vi "AO DM setup.vi"() -> ()   [LabVIEW 2018]
uses:
  <userlib>/WaveKit.lib/Controls/Wavefront Corrector states - ONE.ctl
  <userlib>/WaveKit.lib/Classes/WavefrontCorrector/WavefrontCorrector.lvclass
  <userlib>/WaveKit.lib/Classes/WavefrontCorrectorSet/WavefrontCorrectorSet.lvclass
  <vilib>/Utility/file.llb/Read From Spreadsheet File (DBL).vi
  <vilib>/Analysis/1siggen.llb/Ramp Pattern by Delta.vi
  <userlib>/WaveKit.lib/Classes/ModalCoef/ModalCoef.lvclass
  <userlib>/WaveKit.lib/Controls/Pupil.lvclass
  <vilib>/Analysis/NI_AALBase.lvlib
panel:
  out "DM Status":sgl[](graph)
  in  "SaveFile":bool=TRUE
  in  "Output folder":path=path "D:/Data"
  in  "File prefix name":string="Test"
  out "Final Positions":sgl[](array[numeric])
  out "Zern coef out":sgl[](array[numeric])
  out "Zern index out":i32[](array[numeric])
  in  "Update":bool
  in  "Additional file":path=path "D:/SystemAlignment/system_aberration_20191029.dat"
  in  "Input type":T1(ring)=enum."Zernike Coef"
  in  "Additional Command":bool=TRUE
  in  "Initial offset":bool=TRUE
  in  "Hasao configuration file":path=path "C:/Program Files (x86)/Imagine Optic/Configuration Files/HASO3_first_7364.dat"
  in  "interaction matrix file":path=path "D:/SystemAlignment/IM_20200206.aomi"
  in  "Initial haso file":path=path "D:/SystemAlignment/system_aberration_residual_20191015.has"
  in  "Zern index in":i32[](array[numeric])
  in  "Zern coef in":sgl[](array[numeric])
  out "error out":errorcluster
  out "Initial Positions":sgl[](array[numeric])
  out "Initial State":T2[](array[typedef])
  out "ActuatorsNumber":i32
  in  "error in (no error)":errorcluster
  in  "Offset command file":path=path "D:/SystemAlignment/system_aberration_20200206.dat"
  in  "DM configuration file":path=path "C:/Program Files (x86)/Imagine Optic/Configuration Files/WaveFrontCorrector_mirao52-e_0326.dat"
  in  "stop":bool
  # "Configuration files"
  # "Commands"
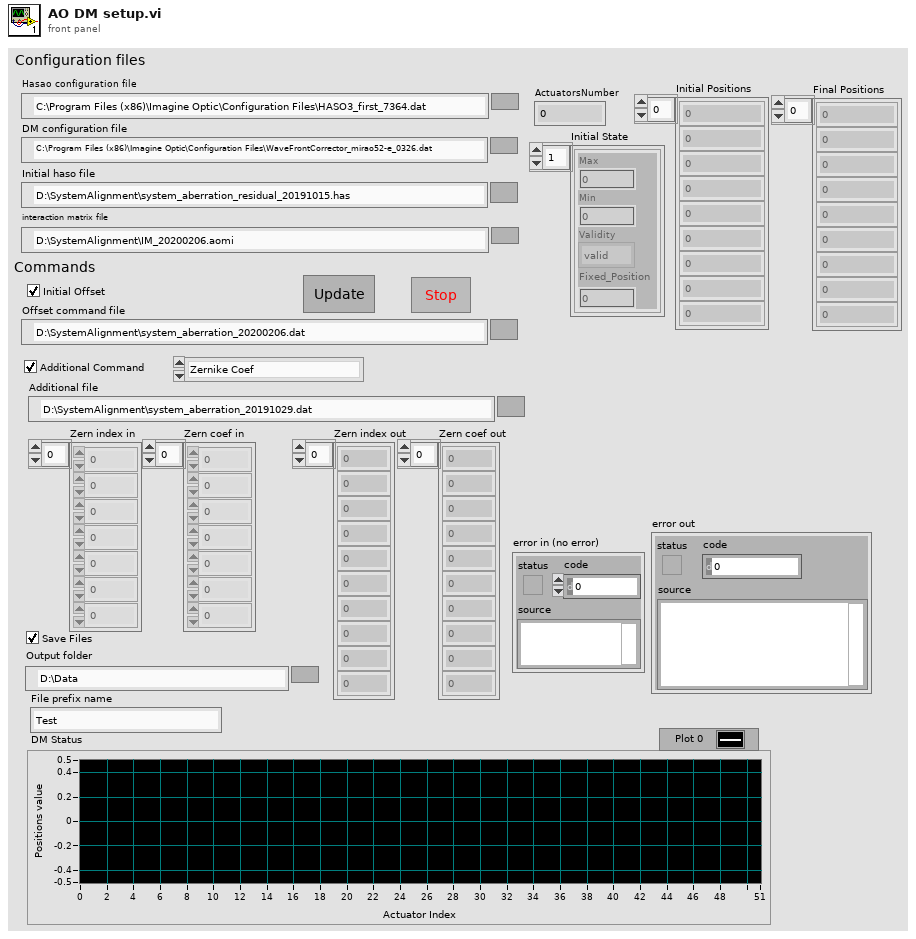
[diagram p1: front panel]
types:
  T1 = enum16{"Zero Input", "Command File", "Zernike Coef", "Zernike File"}
  T2 = typedef "Wavefront Corrector states - ONE.ctl" = cluster{"Max":sgl, "Min":sgl, "Validity":enum16{"valid", "fixed", "invalid"}, "Fixed_Position":sgl}
  T3 = typedef "Wavefront Corrector Position.ctl" = sgl[]
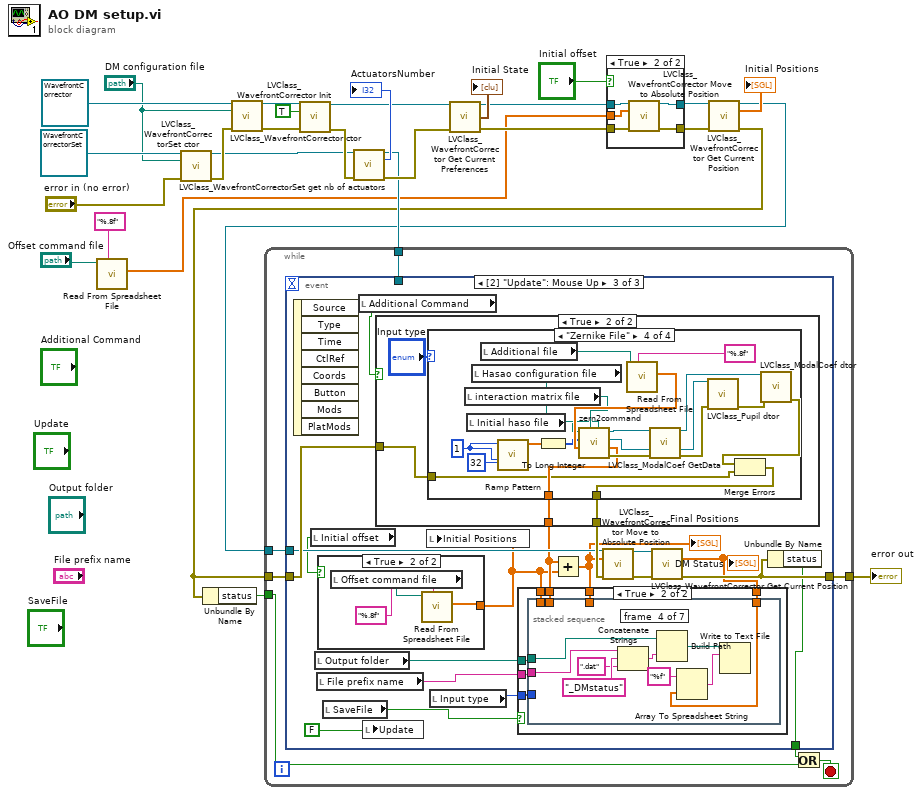
[diagram p0: block diagram]
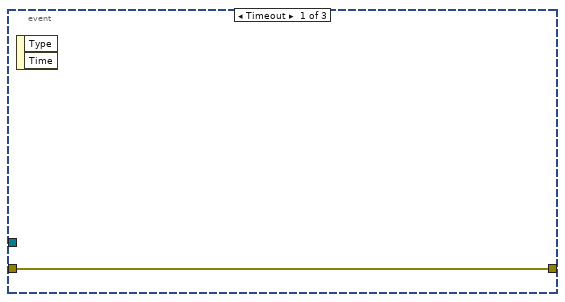
[diagram p3: hidden frame]
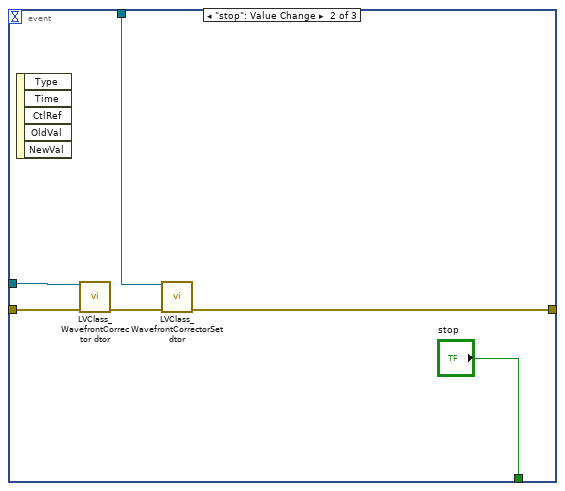
[diagram p4: hidden frame]
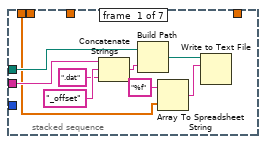
[diagram p6: hidden frame]
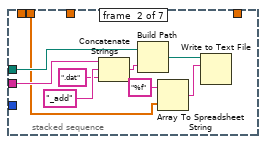
[diagram p7: hidden frame]
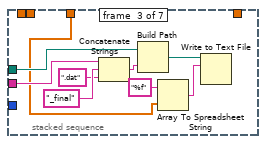
[diagram p8: hidden frame]
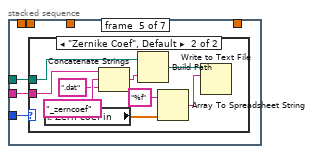
[diagram p9: hidden frame]
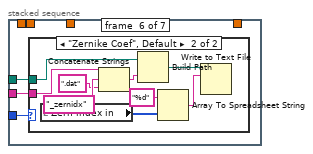
[diagram p11: hidden frame]
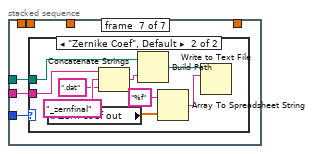
[diagram p13: hidden frame]
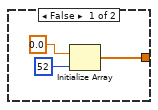
[diagram p15: hidden frame]
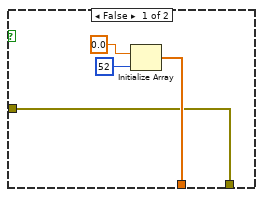
[diagram p16: hidden frame]
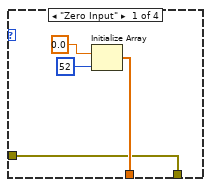
[diagram p17: hidden frame]
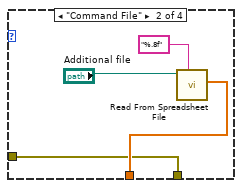
[diagram p18: hidden frame]
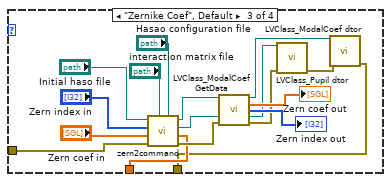
[diagram p19: hidden frame]
diagram:
  n1 = call-poly <vilib>:"Read From Spreadsheet File.vi"("format (%.3f)"="%.8f", "file path (dialog if empty)"="Offset command file") -> ("first row"=w1:dbl[])  [unwired: 5 in, 4 out]
  n2 = call <userlib>:"LVClass_WavefrontCorrectorSet ctor.vi"("WavefrontCorrectorSet in"=refnum<class "WavefrontCorrectorSet.lvclass"> refnum, "PathToWavefrontCorrectorSetupFile"="DM configuration file", "error in (no error)"="error in (no error)") -> ("WavefrontCorrectorSet out"=w15:refnum<class "WavefrontCorrectorSet.lvclass">, "error out"=w24:errorcluster)  [unwired: 11 in]
  n3 = call <userlib>:"LVClass_WavefrontCorrector ctor.vi"("WavefrontCorrector in"=refnum<class "WavefrontCorrector.lvclass"> refnum, "PathToWavefrontCorrectorSetupFile"="DM configuration file", "error in (no error)"=w24) -> ("WavefrontCorrector out"=w19:refnum<class "WavefrontCorrector.lvclass">, "error out"=w18:errorcluster)  [unwired: 11 in]
  n4 = call <userlib>:"LVClass_WavefrontCorrector Init.vi"("WavefrontCorrector in"=w19, "set_init_state_from_config_file"=TRUE, "error in (no error)"=w18) -> ("WavefrontCorrector out"=w13:refnum<class "WavefrontCorrector.lvclass">, "error out"=w17:errorcluster)  [unwired: 11 in]
  n5 = call <userlib>:"LVClass_WavefrontCorrectorSet get nb of actuators.vi"("WavefrontCorrectorSet in"=w15, "error in (no error)"=w17) -> ("WavefrontCorrectorSet out"=w8:refnum<class "WavefrontCorrectorSet.lvclass">, "ActuatorsNumber"=→"ActuatorsNumber":i32, "error out"=w14:errorcluster)  [unwired: 11 in]
  n6 = call <userlib>:"LVClass_WavefrontCorrector Get Current Preferences.vi"("WavefrontCorrector in"=w13, "error in (no error)"=w14) -> ("WavefrontCorrector out"=w5:refnum<class "WavefrontCorrector.lvclass">, "Mirror preferences.Wavefront Corrector State"=→"Initial State":T2[], "error out"=w4:errorcluster)  [unwired: 10 in, 1 out]
  n7 = case shown="True" "Initial offset" {
    tunnel: w1 -> [_ w35]
    tunnel: [w30 w34] -> w10
    tunnel: [w29 w33] -> w9
    tunnel: w5 -> [w30 w32]
    tunnel: w4 -> [w29 w31]
    frame False {
    }
    frame True {
      n8 = call <userlib>:"LVClass_WavefrontCorrector Move to Absolute Position.vi"("WavefrontCorrector in"=w32, "Absolute Positions"=w35, "error in (no error)"=w31) -> ("WavefrontCorrector out"=w34:refnum<class "WavefrontCorrector.lvclass">, "error out"=w33:errorcluster)  [unwired: 11 in]
    }
  }
  n9 = call <userlib>:"LVClass_WavefrontCorrector Get Current Position.vi"("WavefrontCorrector in"=w10, "error in (no error)"=w9) -> ("WavefrontCorrector out"=w2:refnum<class "WavefrontCorrector.lvclass">, "Wavefront Corrector Position"=→"Initial Positions":T3, "error out"=w7:errorcluster)  [unwired: 11 in]
  n10 = Unbundle By Name(w7) -> ("status"=w27:bool)
  n11 = while {
    tunnel: w27 -> [w41]
    tunnel: w8 -> [w39]
    tunnel: w2 -> [w38]
    tunnel: w7 -> [w37]
    tunnel: [w36] -> w6
    stop <- w40 stop-if-true
    n12 = event shown="[2] \"Update\": Mouse Up" {
      selector: _ -> [_ _ _]
      dyn-events: _ -> [_ _ _]
      timeout: _ -> [_ _ _]
      tunnel: [_ "stop" w64] -> w42
      tunnel: w39 -> [_ w48 _]
      tunnel: w38 -> [_ w47 w60]
      tunnel: w37 -> [w43 w46 w67]
      tunnel: [w43 w44 w65] -> w36
      event Timeout {
        n13 = event-data() -> ()  [unwired: 1 in, 2 out]
      }
      event "stop": Value Change {
        n14 = event-data() -> ()  [unwired: 1 in, 5 out]
        n15 = call <userlib>:"LVClass_WavefrontCorrector dtor.vi"("WavefrontCorrector in"=w47, "error in (no error)"=w46) -> ("error out"=w45:errorcluster)  [unwired: 12 in, 1 out]
        n16 = call <userlib>:"LVClass_WavefrontCorrectorSet dtor.vi"("WavefrontCorrectorSet in"=w48, "error in (no error)"=w45) -> ("error out"=w44:errorcluster)  [unwired: 12 in, 1 out]
      }
      event "Update": Mouse Up {
        n17 = event-data() -> ()  [unwired: 1 in, 8 out]
        n18 = local read "Initial offset"() -> (w59:bool)
        n19 = local read "Output folder"() -> (w57:path)
        n20 = local read "File prefix name"() -> (w56:string)
        n21 = case shown="True" w59 {
          tunnel: [w147 w152] -> w52
          frame False {
            n22 = Initialize Array(0.0, 52) -> (w147:dbl[])
          }
          frame True {
            n23 = local read "Offset command file"() -> (w151:path)
            n24 = call-poly <vilib>:"Read From Spreadsheet File.vi"("format (%.3f)"="%.8f", "file path (dialog if empty)"=w151) -> ("first row"=w152:dbl[])  [unwired: 5 in, 4 out]
          }
        }
        n25 = local read "SaveFile"() -> (w58:bool)
        n26 = local read "Additional Command"() -> (w66:bool)
        n27 = local write "Update"(FALSE ("left")) -> ()
        n28 = case shown="True" w66 {
          tunnel: w67 -> [w153 w160]
          tunnel: [w154 w158] -> w55
          tunnel: [w153 w157] -> w61
          frame False {
            n29 = Initialize Array(0.0, 52) -> (w154:dbl[])
          }
          frame True {
            n30 = case shown="\"Zernike File\"" "Input type" {
              tunnel: w160 -> [w161 w165 w172 w187]
              tunnel: [w162 w166 w170 w189] -> w158
              tunnel: [w161 w165 w169 w186] -> w157
              frame "Zero Input" {
                n31 = Initialize Array(0.0, 52) -> (w162:dbl[])
              }
              frame "Command File" {
                n32 = call-poly <vilib>:"Read From Spreadsheet File.vi"("format (%.3f)"="%.8f", "file path (dialog if empty)"="Additional file") -> ("first row"=w166:dbl[])  [unwired: 5 in, 4 out]
              }
              frame "Zernike Coef", Default {
                n33 = call "zern2command.vi"("Hasao configuration file"="Hasao configuration file", "interaction matrix file"="interaction matrix file", "error in (no error)"=w172, "Zern coef in"="Zern coef in", "Zern index in"="Zern index in", "Initial haso file"="Initial haso file") -> ("error out"=w171:errorcluster, "Offset Positions"=w170:sgl[], "Zern pupil out"=w173:refnum<class "Pupil.lvclass">, "ModalCoef out"=w174:refnum<class "ModalCoef.lvclass">)  [unwired: 2 in]
                n34 = call <userlib>:"LVClass_ModalCoef GetData.vi"("ModalCoef in"=w174, "Pupil.lvclass"=w173, "error in (no error)"=w171) -> ("ModalCoef out"=w180:refnum<class "ModalCoef.lvclass">, "coef"=→"Zern coef out":sgl[], "index"=→"Zern index out":u32[], "Pupil.lvclass (dup)"=w177:refnum<class "Pupil.lvclass">, "error out"=w176:errorcluster)  [unwired: 8 in]
                n35 = call <userlib>:"LVClass_Pupil dtor.vi"("Pupil in"=w177, "error in (no error)"=w176) -> ("error out"=w175:errorcluster)  [unwired: 12 in, 1 out]
                n36 = call <userlib>:"LVClass_ModalCoef dtor.vi"("ModalCoef in"=w180, "error in (no error)"=w175) -> ("error out"=w169:errorcluster)  [unwired: 12 in, 1 out]
              }
              frame "Zernike File" {
                w192 = 1
                n37 = local read "interaction matrix file"() -> (w196:path)
                n38 = local read "Initial haso file"() -> (w194:path)
                n39 = local read "Hasao configuration file"() -> (w195:path)
                n40 = local read "Additional file"() -> (w205:path)
                n41 = call-poly <vilib>:"Ramp Pattern.vi"("start"=w192, "end"=32, "delta"=w192) -> ("Ramp Pattern"=w193:dbl[])  [unwired: 6 in, 2 out]
                n42 = To Long Integer(number=w193) -> (32bit integer=w190:i32[])
                n43 = call-poly <vilib>:"Read From Spreadsheet File.vi"("format (%.3f)"="%.8f", "file path (dialog if empty)"=w205) -> ("first row"=w197:dbl[])  [unwired: 5 in, 4 out]
                n44 = call "zern2command.vi"("Hasao configuration file"=w195, "interaction matrix file"=w196, "Zern coef in"=w197, "Zern index in"=w190, "Initial haso file"=w194) -> ("error out"=w198:errorcluster, "Offset Positions"=w189:sgl[], "Zern pupil out"=w199:refnum<class "Pupil.lvclass">, "ModalCoef out"=w200:refnum<class "ModalCoef.lvclass">)  [unwired: 3 in]
                n45 = call <userlib>:"LVClass_ModalCoef GetData.vi"("ModalCoef in"=w200, "Pupil.lvclass"=w199, "error in (no error)"=w198) -> ("ModalCoef out"=w204:refnum<class "ModalCoef.lvclass">, "Pupil.lvclass (dup)"=w203:refnum<class "Pupil.lvclass">, "error out"=w202:errorcluster)  [unwired: 8 in, 2 out]
                n46 = call <userlib>:"LVClass_Pupil dtor.vi"("Pupil in"=w203, "error in (no error)"=w202) -> ("error out"=w201:errorcluster)  [unwired: 12 in, 1 out]
                n47 = call <userlib>:"LVClass_ModalCoef dtor.vi"("ModalCoef in"=w204, "error in (no error)"=w201) -> ("error out"=w188:errorcluster)  [unwired: 12 in, 1 out]
                n48 = Merge Errors(w188, w187) -> (w186:errorcluster)
              }
            }
          }
        }
        n49 = local write "Initial Positions"(w52) -> ()
        n50 = local read "Input type"() -> (w54:T1)
        n51 = Add(x=w55, y=w52) -> (x+y=w53:dbl[])
        "Final Positions" <- w53
        n52 = call <userlib>:"LVClass_WavefrontCorrector Move to Absolute Position.vi"("WavefrontCorrector in"=w60, "Absolute Positions"=w53, "error in (no error)"=w61) -> ("WavefrontCorrector out"=w62:refnum<class "WavefrontCorrector.lvclass">, "error out"=w63:errorcluster)  [unwired: 11 in]
        n53 = call <userlib>:"LVClass_WavefrontCorrector Get Current Position.vi"("WavefrontCorrector in"=w62, "error in (no error)"=w63) -> ("Wavefront Corrector Position"=w50:T3, "error out"=w65:errorcluster)  [unwired: 11 in, 1 out]
        "DM Status" <- w50
        n54 = case shown="True" w58 {
          tunnel: w57 -> [_ w74]
          tunnel: w56 -> [_ w73]
          tunnel: w52 -> [_ w72]
          tunnel: w55 -> [_ w71]
          tunnel: w53 -> [_ w70]
          tunnel: w54 -> [_ w69]
          tunnel: w50 -> [_ w68]
          frame False {
          }
          frame True {
            n55 = stacked-sequence {
              tunnel: w74 -> [w79 w88 w97 w106 w113 w125 w137]
              tunnel: w73 -> [w77 w86 w95 w104 w112 w124 w136]
              tunnel: w72 -> [w75 _ _ _ _ _ _]
              tunnel: w71 -> [_ w84 _ _ _ _ _]
              tunnel: w70 -> [_ _ w93 _ _ _ _]
              tunnel: w69 -> [_ _ _ _ w111 w123 w135]
              tunnel: w68 -> [_ _ _ w102 _ _ _]
              frame #0 {
                n56 = Concatenate Strings(w77, "_offset", ".dat") -> (w80:string)
                n57 = Build Path(base path=w79, name or relative path=w80) -> (appended path=w81:path)
                n58 = Array To Spreadsheet String(array=w75, 3:"%f") -> (spreadsheet string=w82:string)  [unwired: 1 in]
                n59 = Write to Text File(file (use dialog)=w81, text=w82) -> ()  [unwired: 2 in, 3 out]
              }
              frame #1 {
                n60 = Concatenate Strings(w86, "_add", ".dat") -> (w89:string)
                n61 = Build Path(base path=w88, name or relative path=w89) -> (appended path=w90:path)
                n62 = Array To Spreadsheet String(array=w84, 3:"%f") -> (spreadsheet string=w91:string)  [unwired: 1 in]
                n63 = Write to Text File(file (use dialog)=w90, text=w91) -> ()  [unwired: 2 in, 3 out]
              }
              frame #2 {
                n64 = Concatenate Strings(w95, "_final", ".dat") -> (w98:string)
                n65 = Build Path(base path=w97, name or relative path=w98) -> (appended path=w99:path)
                n66 = Array To Spreadsheet String(array=w93, 3:"%f") -> (spreadsheet string=w100:string)  [unwired: 1 in]
                n67 = Write to Text File(file (use dialog)=w99, text=w100) -> ()  [unwired: 2 in, 3 out]
              }
              frame #3 {
                n68 = Concatenate Strings(w104, "_DMstatus", ".dat") -> (w107:string)
                n69 = Build Path(base path=w106, name or relative path=w107) -> (appended path=w108:path)
                n70 = Array To Spreadsheet String(array=w102, 3:"%f") -> (spreadsheet string=w109:string)  [unwired: 1 in]
                n71 = Write to Text File(file (use dialog)=w108, text=w109) -> ()  [unwired: 2 in, 3 out]
              }
              frame #4 {
                n72 = case shown="\"Zernike Coef\", Default" w111 {
                  tunnel: w113 -> [_ w118]
                  tunnel: w112 -> [_ w116]
                  frame "Zero Input" {
                  }
                  frame "Zernike Coef", Default {
                    n73 = local read "Zern coef in"() -> (w114:sgl[])
                    n74 = Concatenate Strings(w116, "_zerncoef", ".dat") -> (w119:string)
                    n75 = Build Path(base path=w118, name or relative path=w119) -> (appended path=w120:path)
                    n76 = Array To Spreadsheet String(array=w114, 3:"%f") -> (spreadsheet string=w121:string)  [unwired: 1 in]
                    n77 = Write to Text File(file (use dialog)=w120, text=w121) -> ()  [unwired: 2 in, 3 out]
                  }
                }
              }
              frame #5 {
                n78 = case shown="\"Zernike Coef\", Default" w123 {
                  tunnel: w125 -> [_ w130]
                  tunnel: w124 -> [_ w128]
                  frame "Zero Input" {
                  }
                  frame "Zernike Coef", Default {
                    n79 = local read "Zern index in"() -> (w126:i32[])
                    n80 = Concatenate Strings(w128, "_zernidx", ".dat") -> (w131:string)
                    n81 = Build Path(base path=w130, name or relative path=w131) -> (appended path=w132:path)
                    n82 = Array To Spreadsheet String(array=w126, 3:"%d") -> (spreadsheet string=w133:string)  [unwired: 1 in]
                    n83 = Write to Text File(file (use dialog)=w132, text=w133) -> ()  [unwired: 2 in, 3 out]
                  }
                }
              }
              frame #6 {
                n84 = case shown="\"Zernike Coef\", Default" w135 {
                  tunnel: w137 -> [_ w142]
                  tunnel: w136 -> [_ w140]
                  frame "Zero Input" {
                  }
                  frame "Zernike Coef", Default {
                    n85 = local read "Zern coef out"() -> (w138:sgl[])
                    n86 = Concatenate Strings(w140, "_zernfinal", ".dat") -> (w143:string)
                    n87 = Build Path(base path=w142, name or relative path=w143) -> (appended path=w144:path)
                    n88 = Array To Spreadsheet String(array=w138, 3:"%f") -> (spreadsheet string=w145:string)  [unwired: 1 in]
                    n89 = Write to Text File(file (use dialog)=w144, text=w145) -> ()  [unwired: 2 in, 3 out]
                  }
                }
              }
            }
          }
        }
        n90 = Unbundle By Name(w65) -> ("status"=w64:bool)
      }
    }
    n91 = Or(x=w42, y=w41) -> (x .or. y?=w40:bool)
  }
  "error out" <- w6
